vi "StopApp Event.vi"(8 "error in (no error)":errorcluster, 11 "EventLog in":refnum<class "EventLog.lvclass">) -> (0 "error out":errorcluster, 3 "Events out":refnum<class "Events.lvclass">)   [LabVIEW 2019, in "Events.lvclass"]
uses:
  Events.lvclass
  SubModules/EventLog/EventLog.lvclass
  Modules/Core/Core/TypeDef/App State.ctl
  Modules/Core/Core/Core.lvclass
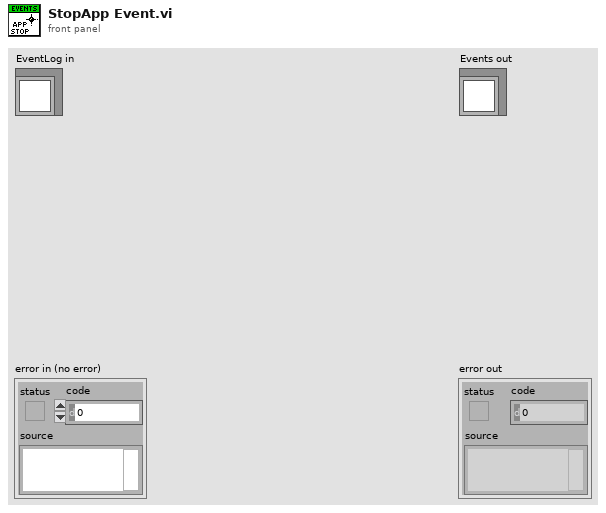
[diagram p1: front panel]
types:
  T1 = typedef "Core.lvlib/Core.lvclass/App State.ctl" = enum16{"Init", "Safe State", "Normal Working", "Closing"}
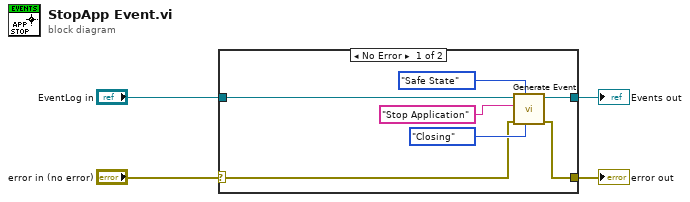
[diagram p0: block diagram]
diagram:
  n1 = case shown="No Error" "error in (no error)" {
    selector: "error in (no error)" -> [w7 w12]
    tunnel: [w6 w12] -> w3
    tunnel: [w11 _] -> w2
    tunnel: "EventLog in" -> [w5 _]
    frame No Error {
      n2 = call "Generate Event.vi"("Next State"=App_State."Closing", "Act State"=App_State."Safe State", "Error In"=w7, "Description"="Stop Application", "EventLog in"=w5) -> ("Error Out"=w6:errorcluster, "Events out"=w11:refnum<class "Events.lvclass">)  [unwired: 5 in]
    }
    frame Error {
    }
  }
  "error out" <- w3
  "Events out" <- w2
